vi "B_ReadWriteClassAttribute.vi"(0 "reference in":refnum<class "BaseTemplate.lvclass">, 5 "Error In":errorcluster) -> (14 "reference out":refnum<class "BaseTemplate.lvclass">, 19 "Error Out":errorcluster)   [LabVIEW 2020, in "BaseTemplate.lvclass"]
uses:
  <resource>/Framework/Providers/Open_GDS/ClassProviders/Provider_EndevoGOOP300/Templates/BaseTemplate/BaseTemplate.lvclass
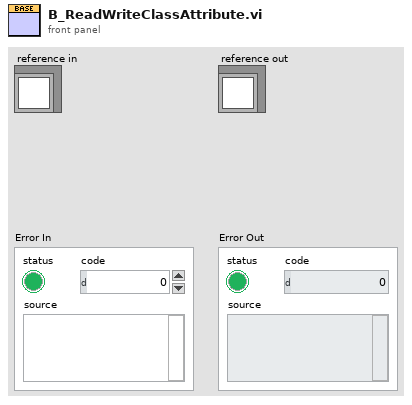
[diagram p1: front panel]
types:
  T1 = typedef "BaseTemplate.lvclass/ClassAttributes.ctl" = cluster{"classAttribute1":bool}
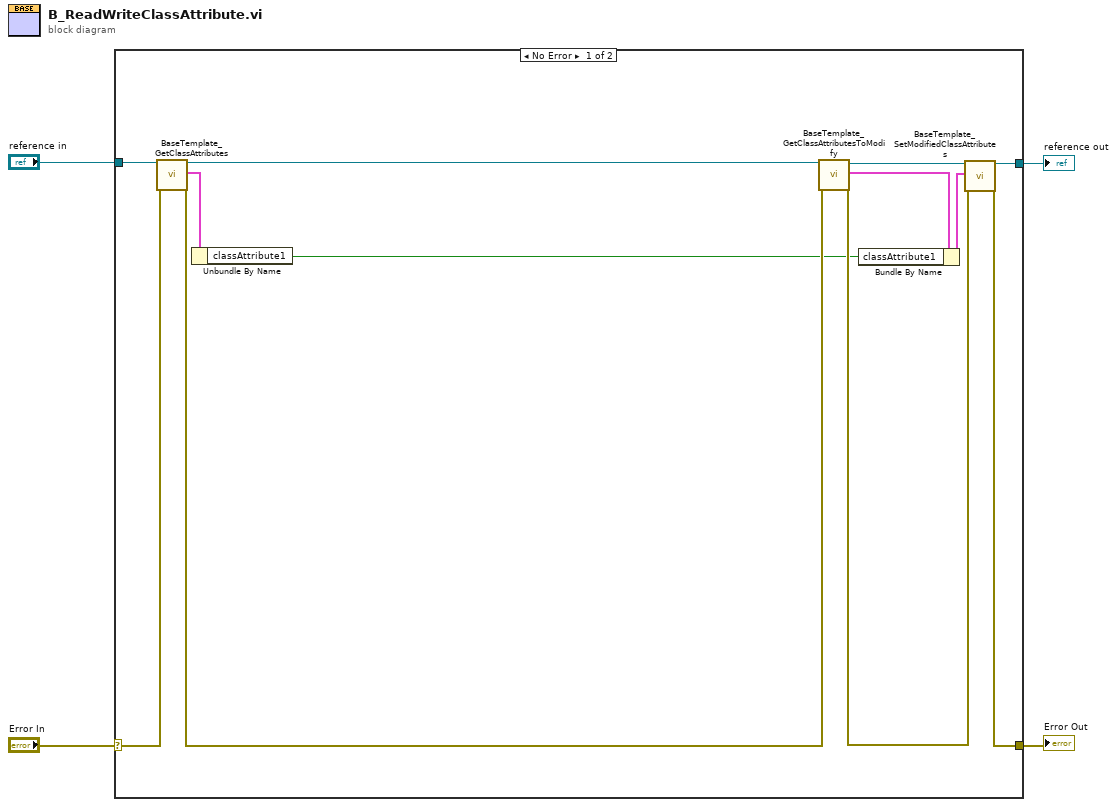
[diagram p0: block diagram]
diagram:
  n1 = case shown="No Error" "Error In" {
    selector: "Error In" -> [w9 w18]
    tunnel: [w13 w18] -> w3
    tunnel: [w12 w17] -> w1
    tunnel: "reference in" -> [w10 w17]
    frame No Error {
      n2 = call <resource>:"BaseTemplate_GetClassAttributes.vi"("reference in"=w10, "error in (no error)"=w9) -> ("reference out"=w7:refnum<class "BaseTemplate.lvclass">, "Class attributes"=w6:T1, "error out"=w8:errorcluster)  [unwired: 14 in, 1 out]
      n3 = Unbundle By Name(w6) -> ("classAttribute1"=w5:bool)
      n4 = call <resource>:"BaseTemplate_GetClassAttributesToModify.vi"("reference in"=w7, "error in (no error)"=w8) -> ("reference out"=w14:refnum<class "BaseTemplate.lvclass">, "Class attributes"=w16:T1, "error out"=w11:errorcluster)  [unwired: 14 in, 1 out]
      n5 = Bundle By Name(cluster=w16, "classAttribute1"=w5) -> (w15:T1)
      n6 = call <resource>:"BaseTemplate_SetModifiedClassAttributes.vi"("reference in"=w14, "Class attributes"=w15, "error in (no error)"=w11) -> ("reference out"=w12:refnum<class "BaseTemplate.lvclass">, "error out"=w13:errorcluster)  [unwired: 15 in]
    }
    frame Error {
    }
  }
  "Error Out" <- w3
  "reference out" <- w1
